vi "MakeBox.vi"(8 "error in (no error)":errorcluster, 10 "Size":i32, 11 "Array in":T1[][](array[typedef])) -> (0 "error out":errorcluster, 3 "Array out":T1[][](array[typedef]))   [LabVIEW 2020]
doc: "Modifies a Board of a given size - adds walls at the borders"
uses:
  TypeDef/tiles-key.ctl
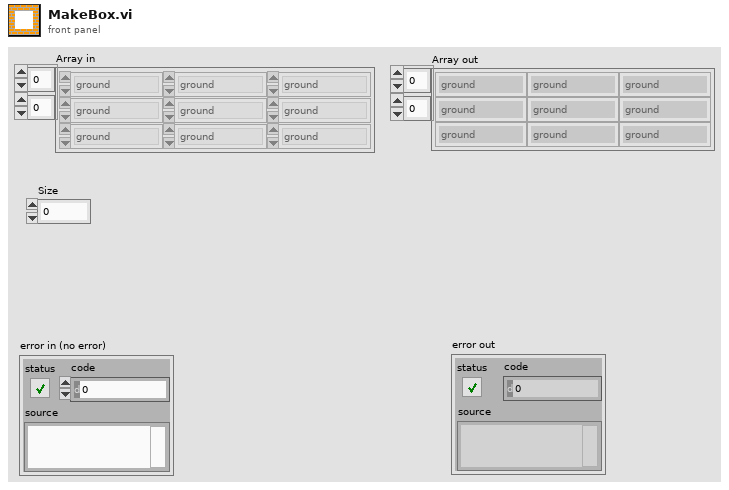
[diagram p1: front panel]
types:
  T1 = typedef "tiles-key.ctl" = enum16{"ground", "wall", "head (right)", "head (up)", "head (left)", "head (down)", "L-turn (right-up)", "L-turn (up-left)", "L-turn (left-down)", "L-turn (down-right)", "body (right)", "body (up)", "body (left)", "body (down)", "R-turn (right-down)", "R-turn (up-right)", "R-turn (left-up)", "R-turn (down-left)", "tail (right)", "tail (up)", "tail (left)", "tail (down)", "dead head (right)", "dead head (up)", "dead head (left)", "dead head (down)", "dead L-turn (right-up)", "dead L-turn (up-left)", "dead L-turn (left-down)", "dead L-turn (down-right)", "dead body (right)", "dead body (up)", "dead body (left)", "dead body (down)", "dead R-turn (right-down)", "dead R-turn (up-right)", "dead R-turn (left-up)", "dead R-turn (down-left)", "dead tail (right)", "dead tail (up)", "dead tail (left)", "dead tail (down)", "target red", "target blue", "target yellow", "target green"}
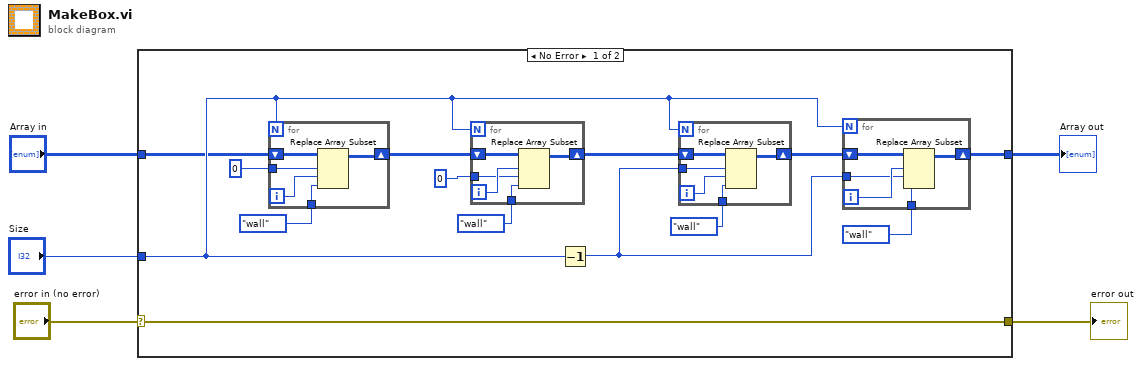
[diagram p0: block diagram]
diagram:
  n1 = case shown="No Error" "error in (no error)" {
    selector: "error in (no error)" -> [w6 w40]
    tunnel: "Size" -> [w19 _]
    tunnel: "Array in" -> [w17 w41]
    tunnel: [w7 w41] -> w3
    tunnel: [w6 w40] -> w1
    frame No Error {
      n2 = for {
        N: w19 -> [_]
        tunnel: 0 -> [w38]
        tunnel: tiles-key."wall" ("Tiles-key") -> [w35]
        shift-right: [w36] -> w14
        shift-left: w17 -> [w39]
        i -> [w37]
        n3 = Replace Array Subset(array=w39, new element=w35, index (row)=w38, index (col)=w37) -> (w36:T1[][])
      }
      n4 = for {
        N: w19 -> [_]
        tunnel: 0 -> [w26]
        tunnel: tiles-key."wall" ("Tiles-key") -> [w25]
        shift-right: [w28] -> w11
        shift-left: w14 -> [w29]
        i -> [w27]
        n5 = Replace Array Subset(array=w29, new element=w25, index (row)=w27, index (col)=w26) -> (w28:T1[][])
      }
      n6 = Decrement(x=w19) -> (x-1=w16:i32)
      n7 = for {
        N: w19 -> [_]
        tunnel: w16 -> [w33]
        tunnel: tiles-key."wall" ("Tiles-key") -> [w30]
        shift-right: [w31] -> w10
        shift-left: w11 -> [w34]
        i -> [w32]
        n8 = Replace Array Subset(array=w34, new element=w30, index (row)=w33, index (col)=w32) -> (w31:T1[][])
      }
      n9 = for {
        N: w19 -> [_]
        tunnel: w16 -> [w21]
        tunnel: tiles-key."wall" ("Tiles-key") -> [w20]
        shift-right: [w22] -> w7
        shift-left: w10 -> [w24]
        i -> [w23]
        n10 = Replace Array Subset(array=w24, new element=w20, index (row)=w23, index (col)=w21) -> (w22:T1[][])
      }
    }
    frame Error {
    }
  }
  "Array out" <- w3
  "error out" <- w1
